vi "Destroy Notifiers.vi"(11 "SCADA Communications in":refnum<class "SCADA Communications.lvclass">) -> (3 "SCADA Communications out":refnum<class "SCADA Communications.lvclass">)   [LabVIEW 2015, in "SCADA Communcations Actor.lvlib" / "SCADA Communications.lvclass"]
uses:
  SCADA Communications.lvclass
  SCADA Communications.lvclass/SCADA Communications.ctl
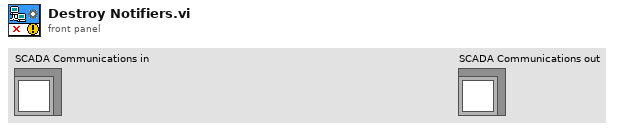
[diagram p1: front panel]
types:
  T1 = typedef "SCADA Communcations Actor.lvlib/SCADA Communications.lvclass/Notifiers Cluster.ctl" = cluster{"stop":refnum<notifier>, "Comms stop":refnum<notifier>}
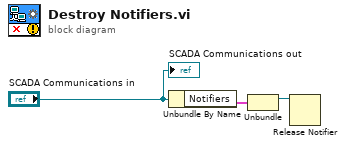
[diagram p0: block diagram]
diagram:
  n1 = Unbundle By Name("SCADA Communications in") -> ("Notifiers"=w3:T1)
  n2 = Unbundle(w3) -> ("stop"=w1:refnum<notifier>)  [unwired: 1 out]
  n3 = Release Notifier(notifier=w1) -> ()  [unwired: 2 in, 3 out]
  "SCADA Communications out" <- "SCADA Communications in"
